vi "Init.vi"(8 "error in (no error)":errorcluster, 9 "state_variables":T1, 10 "model_v1_parameters":T2, 11 "Model_Predictor in":refnum<class "Model_Predictor.lvclass">) -> (0 "error out":errorcluster, 3 "Model_Predictor out":refnum<class "Model_Predictor.lvclass">)   [LabVIEW 2021, in "MBPOnOff_Controller.lvlib" / "Model_Predictor.lvclass"]
uses:
  Model_Predictor.lvclass
  typedefs/Model_v1_parameters.ctl
  typedefs/state_variables.ctl
  OUR_Monitor/OUR_Monitor.lvclass
  Model_Predictor.lvclass/Model_Predictor.ctl
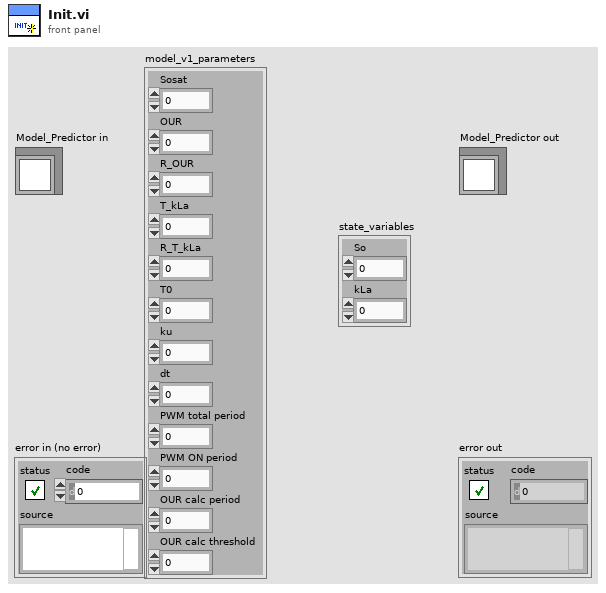
[diagram p1: front panel]
types:
  T1 = typedef "MBPOnOff_Controller.lvlib/Model_Predictor.lvclass/state_variables.ctl" = cluster{"So":dbl, "kLa":dbl}
  T2 = typedef "MBPOnOff_Controller.lvlib/Model_Predictor.lvclass/Model_v1_parameters.ctl" = cluster{"Sosat":dbl, "OUR":dbl, "R_OUR":dbl, "T_kLa":dbl, "R_T_kLa":dbl, "T0":dbl, "ku":dbl, "dt":dbl, "PWM total period":dbl, "PWM ON period":dbl, "OUR calc period":dbl, "OUR calc threshold":dbl}
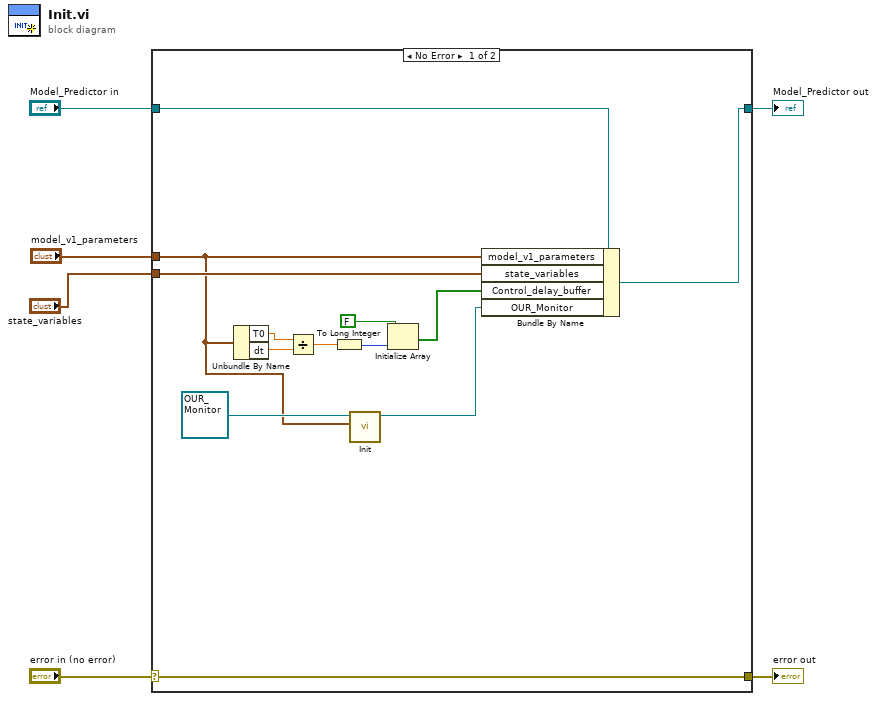
[diagram p0: block diagram]
diagram:
  n1 = case shown="No Error" "error in (no error)" {
    selector: "error in (no error)" -> [w18 w21]
    tunnel: [w18 w21] -> w5
    tunnel: [w17 w20] -> w3
    tunnel: "Model_Predictor in" -> [w19 w20]
    tunnel: "model_v1_parameters" -> [w8 _]
    tunnel: "state_variables" -> [w16 _]
    frame No Error {
      n2 = Unbundle By Name(w8) -> ("T0"=w15:dbl, "dt"=w14:dbl)
      n3 = Divide(x=w15, y=w14) -> (x/y=w13:dbl)
      n4 = To Long Integer(number=w13) -> (32bit integer=w12:i32)
      n5 = call "Init.vi"("model_v1_parameters"=w8, "OUR_Monitor in"=refnum<class "OUR_Monitor.lvclass"> refnum ("MBPOnOff_Controller.lvlib:OUR_Monitor.lvclass")) -> ("OUR_Monitor out"=w7:refnum<class "OUR_Monitor.lvclass">)  [unwired: 8 in, 1 out]
      n6 = Initialize Array(FALSE, w12) -> (w10:bool[])
      n7 = Bundle By Name(cluster=w19, "model_v1_parameters"=w8, "state_variables"=w16, "Control_delay_buffer"=w10, "OUR_Monitor"=w7) -> (w17:refnum<class "Model_Predictor.lvclass">)
    }
    frame Error {
    }
  }
  "error out" <- w5
  "Model_Predictor out" <- w3
